vi "Connection Manager (customizable).vi"(9 "Required":cluster{"DI":string[]}[](array[cluster])=[{"DI"=[]}, {"DI"=[]}, {"DI"=["Rep Trigger", "State Change", "Trial Change"]}, {"DI"=["Rep Trigger", "State Change", "Trial Change"]}], 11 "Configuration file":path=path "C:/ProgramData/EPL/Tosca Defaults.ini") -> (2 "Changed":bool)   [LabVIEW 2020]
uses:
  Type Defs/General PXISlot XControl/PXISlotGP.xctl
  Utility VIs/Controls/KListboxEx/KListboxEx.xctl
  Utility VIs/Controls/KTable/KTable.xctl
  Type Defs/CM-Connection.ctl
  Utility VIs/Controls/KTable/Event Type.ctl
  Utility VIs/File IO VIs/Configuration File Wrapper VIs/Config-Read Key (string).vi
  Utility VIs/File IO VIs/Configuration File Wrapper VIs/Config-Write Key (string).vi
  epl-tosca/LV Source/TTL VIs/Device Classes/Base Class/TTLControlledDevice.lvclass
  epl-tosca/LV Source/TTL VIs/Typedefs/TTLControlledDevice XControl/TTLControlledDevice.xctl
  D:/Development/epl-vi-lib/Koop/KObject Class/KObject.lvclass
  D:/Development/epl-tosca/LV Source/TTL VIs/Device Classes/Base Class/TTLControlledDevice.lvclass
  epl-tosca/LV Source/TTL VIs/Device Classes/WaterDelivery Class/TTLWaterDelivery.lvclass
panel:
  in  "Show effectors":bool
  in  "DE List":i32(xcontrol)
  out "read config":bool=TRUE
  in  "DI List":i32(xcontrol) caption="Inputs"
  in  "DO List":i32(xcontrol) caption="Outputs"
  in  "AI List":i32(xcontrol) caption="Inputs"
  in  "AO List":i32(xcontrol)=1 caption="Outputs"
  in  "Apply Button":bool
  in  "Show digital":bool
  in  "Show analog":bool
  out "Save Op":enum16{"None", "Save", "Save and Exit"}(ring)
  in  "Hide unused":bool
  in  "Exit":bool
  in  "Tab Control":enum32{"Analog", "Digital", "Effectors"}(tab)=enum."Effectors"
  in  "Conn2":cluster{"Outputs":string[], "Inputs":string[]}(xcontrol)={"Outputs"=["", ""], "Inputs"=["", "", "", "", "", "", "", ""]} caption="Slot -1"
  in  "Conn1":cluster{"Outputs":string[], "Inputs":string[]}(xcontrol)={"Outputs"=["", ""], "Inputs"=["", ""]} caption="Slot -1"
  in  "Conn3":cluster{"Outputs":string[], "Inputs":string[]}(xcontrol)={"Outputs"=["Fuck", "Freefield"], "Inputs"=["", "", "", "", "", "", "", ""]} caption="Slot -1"
  in  "Conn4":cluster{"Outputs":string[], "Inputs":string[]}(xcontrol)={"Outputs"=["", "", "", ""], "Inputs"=["", "", "", "", "", "", "", ""]} caption="Slot -1"
  in  "Conn5":cluster{"Outputs":string[], "Inputs":string[]}(xcontrol) caption="Slot -1"
  in  "DO Port":u16(ring)=7 caption="Digital Output Port" items=["PXI1Slot6/port0", "PXI1Slot6/port1", "PXI1Slot6/port2", "PXI1Slot7/port0", "PXI1Slot7/port1", "PXI1Slot7/port2", "PXI1Slot8/port0", "PXI1Slot8/port1", "PXI1Slot8/port2"]
  in  "DI Port":u16(ring)=6 caption="Digital Input Port" items=["PXI1Slot6/port0", "PXI1Slot6/port1", "PXI1Slot6/port2", "PXI1Slot7/port0", "PXI1Slot7/port1", "PXI1Slot7/port2", "PXI1Slot8/port0", "PXI1Slot8/port1", "PXI1Slot8/port2"]
  in  "DO Table":u16(xcontrol)
  in  "DI Table":u16(xcontrol)
  in  "DigDevice 4":refnum<class "TTLControlledDevice.lvclass">(xcontrol)
  in  "DigDevice 3":refnum<class "TTLControlledDevice.lvclass">(xcontrol)
  in  "DigDevice 2":refnum<class "TTLControlledDevice.lvclass">(xcontrol)
  in  "DigDevice 1":refnum<class "TTLControlledDevice.lvclass">(xcontrol)=refnum
  in  "DigDevice 0":refnum<class "TTLControlledDevice.lvclass">(xcontrol)=refnum
  # "ANALOG"
  # "DIGITAL"
  # "TTL-Controlled Devices"
  # "DIGITAL"
  # "TTL-Controlled Devices"
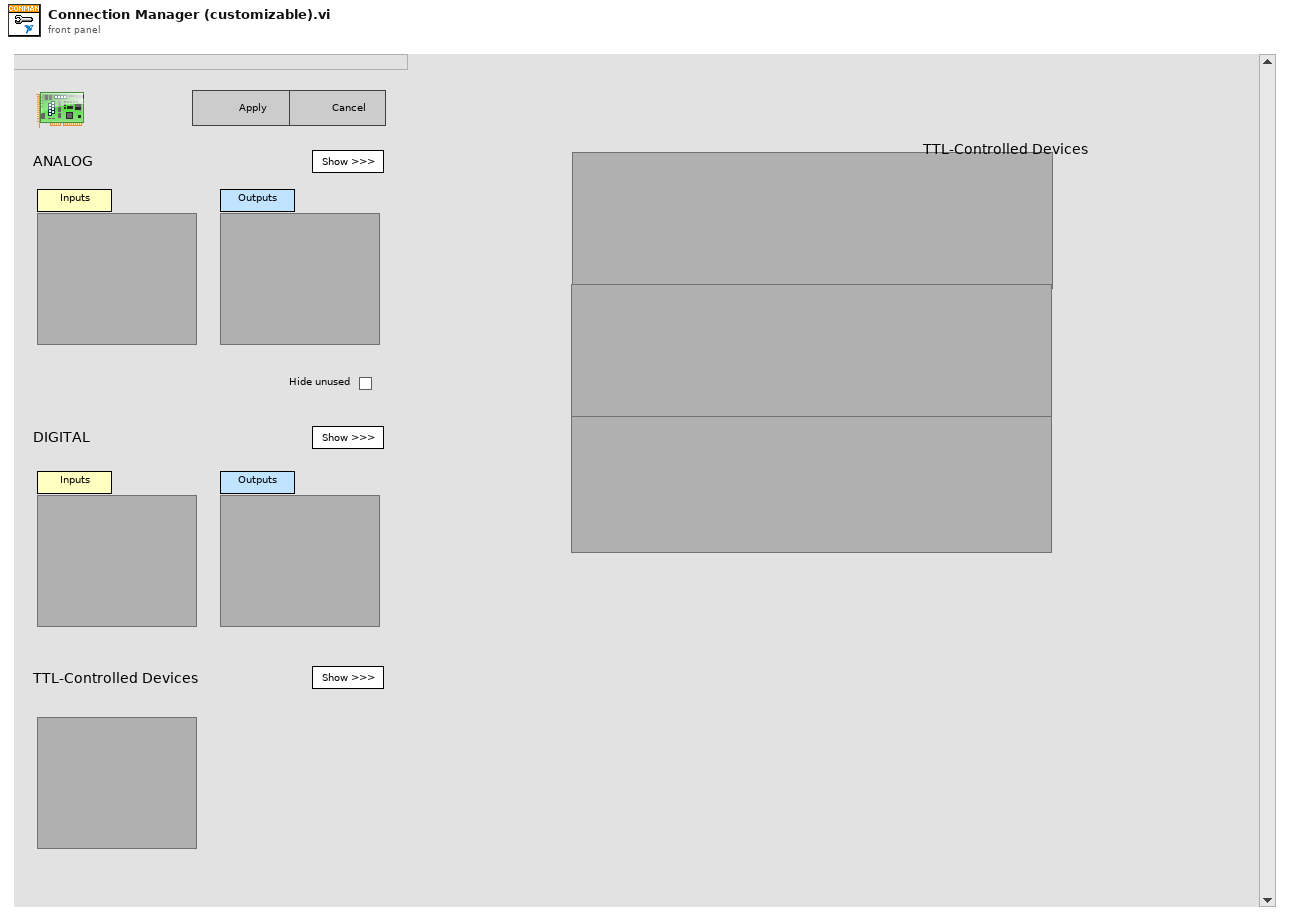
[diagram p1: front panel]
types:
  T1 = typedef "CM-Connection.ctl" = cluster{"IOChannel":string, "Endpoint":string}
  T2 = typedef "KTable.xctl/Event Type.ctl" = enum16{"None", "Selection", "Edit", "Insert", "Delete", "Up", "Down", "Duplicate"}
  T3 = typedef "PXI-Device Spec.ctl" = cluster{"Slot":i32, "ProductType":string, "NumAO":i32, "NumAI":i32, "Device Name":string}
  T4 = cluster{"AO Endpoints":string[], "AI Endpoints":string[]}[]
  T5 = typedef "Connector Type.ctl" = enum16{"None", "PXI-4461", "BNC-2110", "BNC-2090", "PXIe-4463", "PXIe-4464"}
  T6 = typedef "KListboxEx.xctl/Event Action.ctl" = enum16{"None", "Add", "Delete", "Move", "Edit", "Select"}
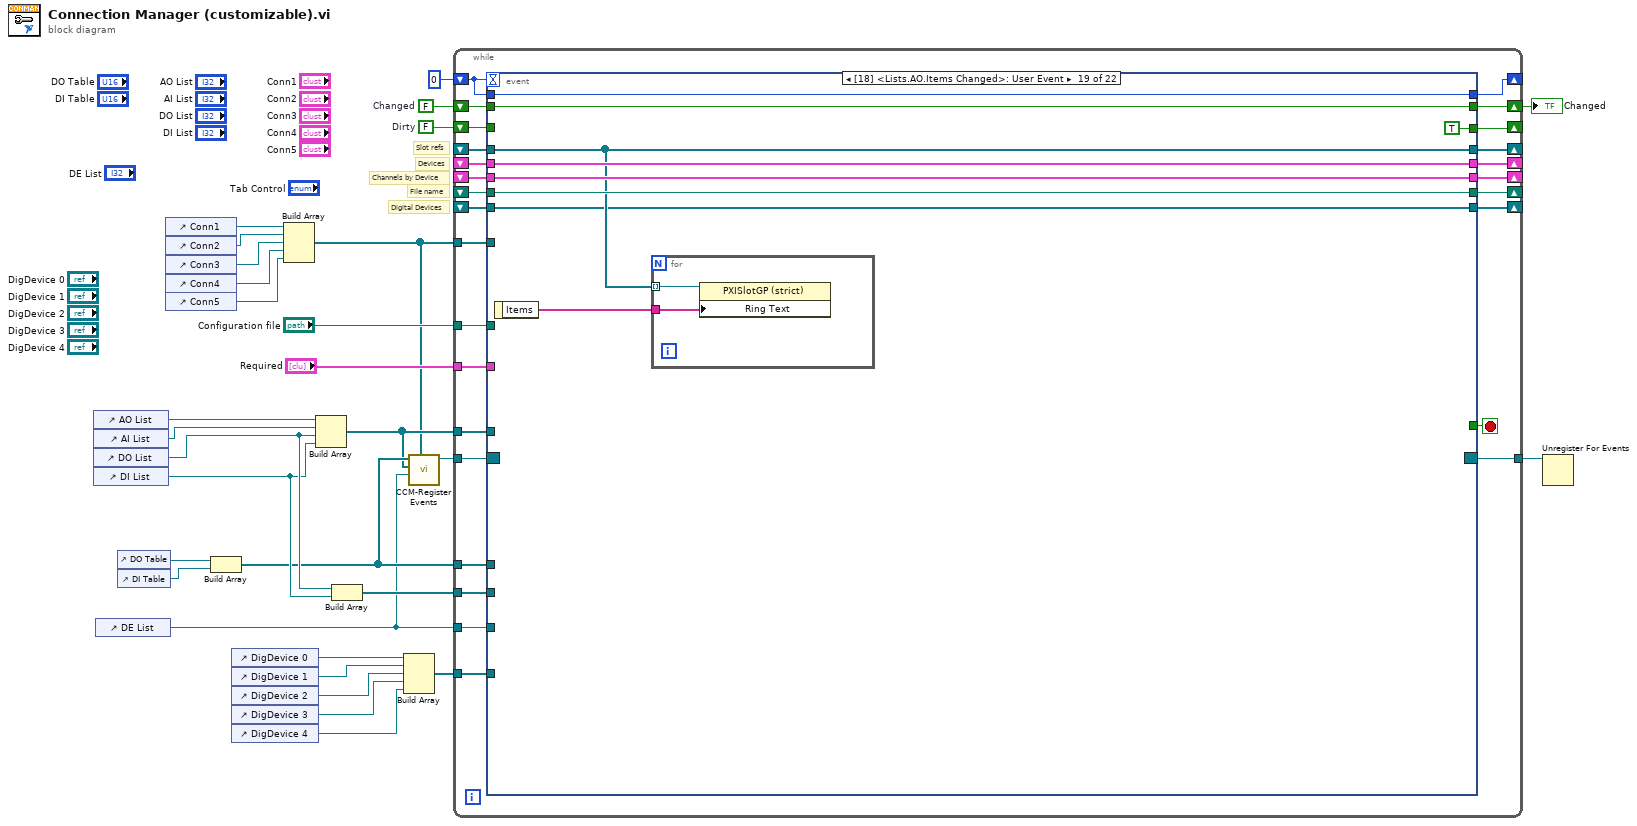
[diagram p0: block diagram]
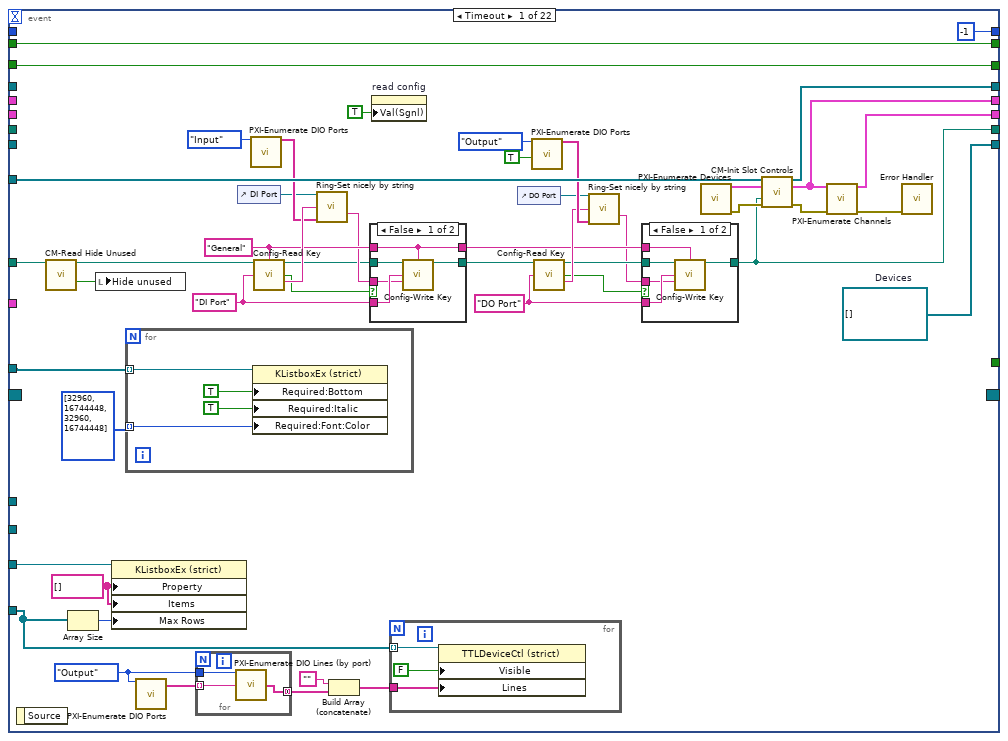
[diagram p2: hidden frame]
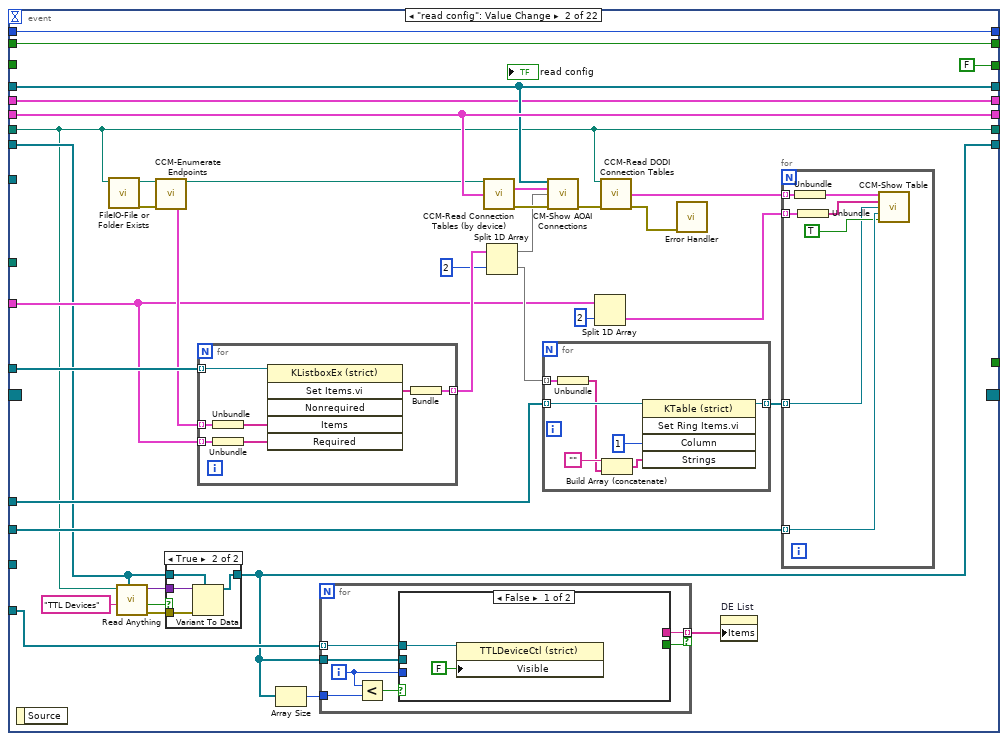
[diagram p5: hidden frame]
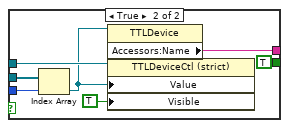
[diagram p6: hidden frame]
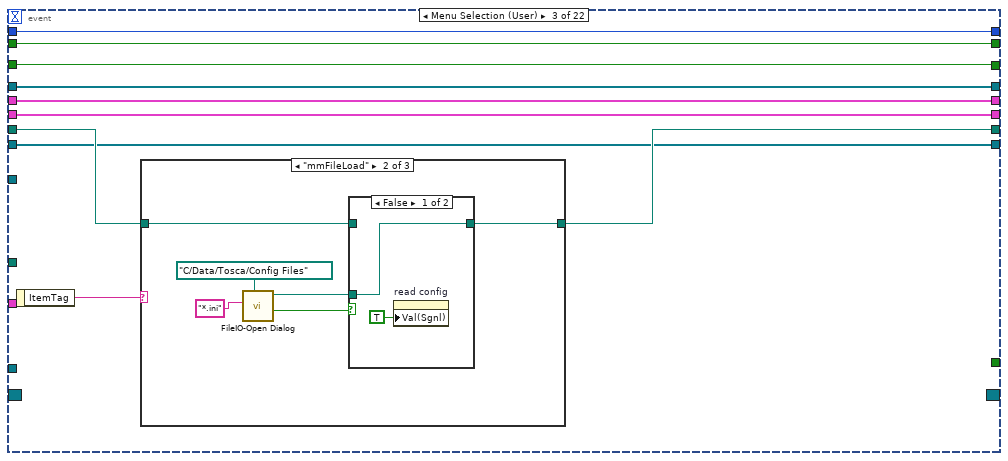
[diagram p8: hidden frame]
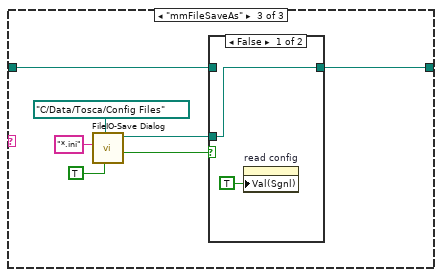
[diagram p11: hidden frame]
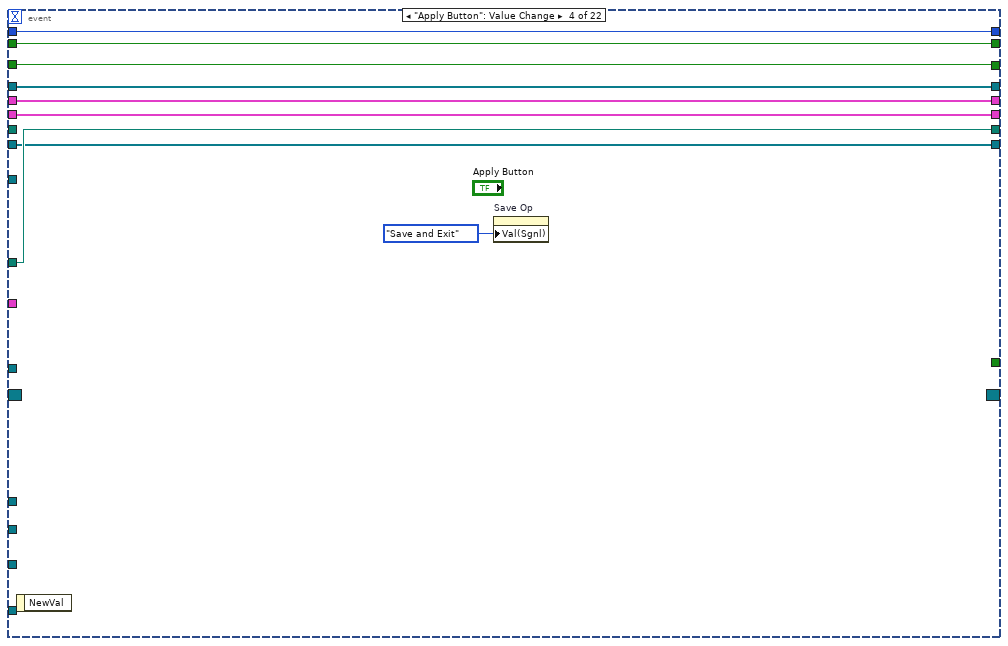
[diagram p13: hidden frame]
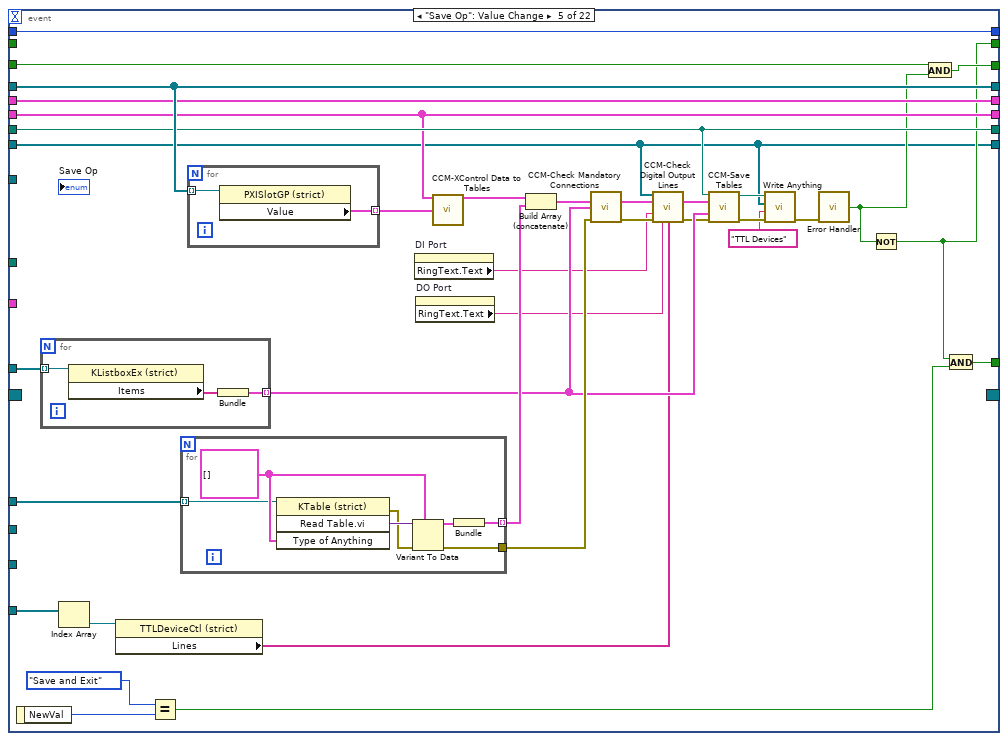
[diagram p14: hidden frame]
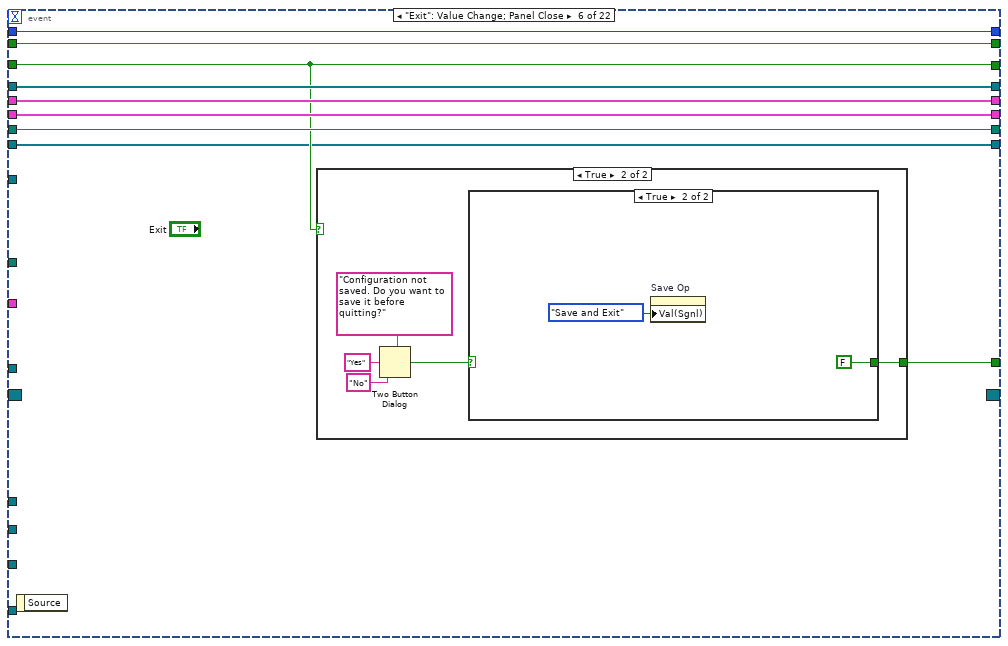
[diagram p15: hidden frame]
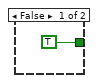
[diagram p16: hidden frame]
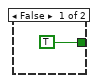
[diagram p17: hidden frame]
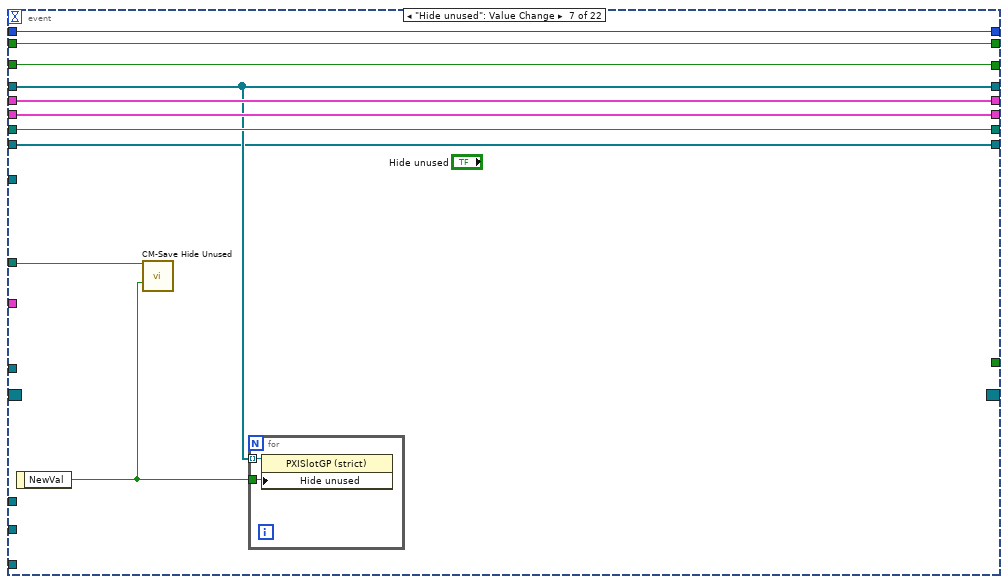
[diagram p18: hidden frame]
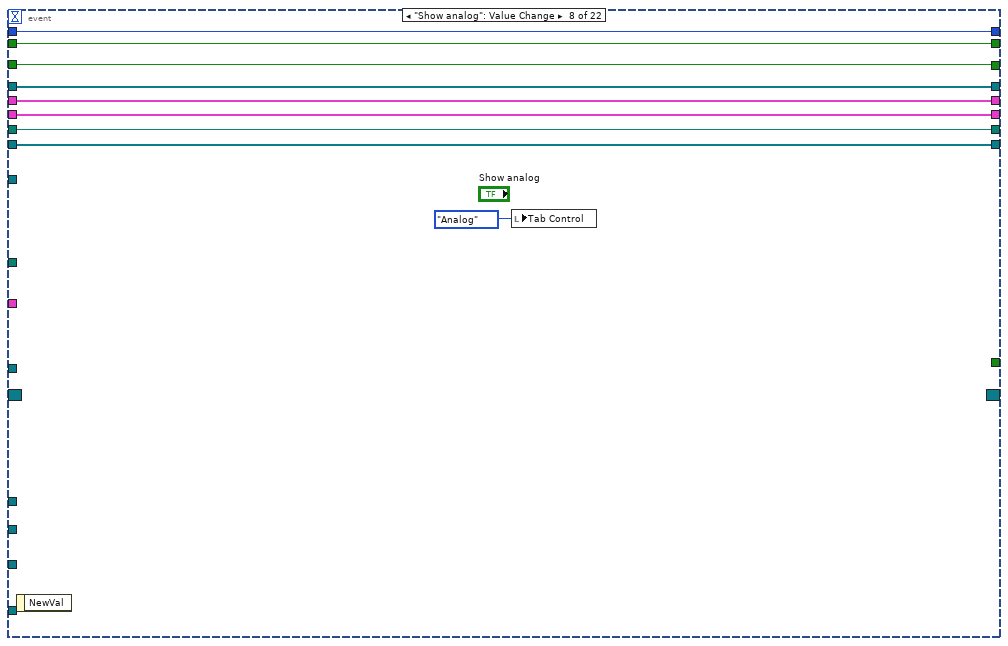
[diagram p19: hidden frame]
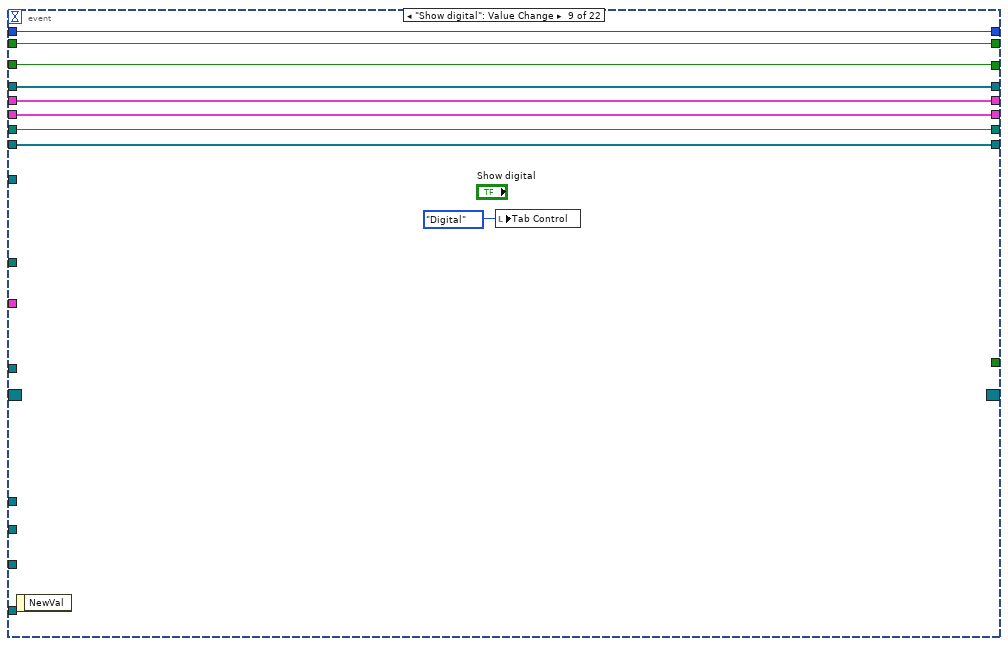
[diagram p20: hidden frame]
diagram:
  w20 = FALSE  # Changed
  w23 = FALSE  # Dirty
  # "Digital Devices"
  # "File name"
  # "Channels by Device"
  # "Devices"
  # "Slot refs"
  n1 = control-ref of="AO List"() -> (w22:refnum<vi>)
  n2 = control-ref of="AI List"() -> (w21:refnum<vi>)
  n3 = control-ref of="DO List"() -> (w19:refnum<vi>)
  n4 = control-ref of="DI List"() -> (w18:refnum<vi>)
  n5 = control-ref of="DE List"() -> (w7:refnum<vi>)
  n6 = control-ref of="DO Table"() -> (w16:refnum<vi>)
  n7 = control-ref of="DI Table"() -> (w15:refnum<vi>)
  n8 = control-ref of="Conn1"() -> (w26:refnum<vi>)
  n9 = control-ref of="Conn2"() -> (w27:refnum<vi>)
  n10 = control-ref of="Conn3"() -> (w28:refnum<vi>)
  n11 = control-ref of="Conn4"() -> (w25:refnum<vi>)
  n12 = control-ref of="Conn5"() -> (w24:refnum<vi>)
  n13 = Build Array(w16, w15) -> (w13:refnum<vi>[])
  n14 = control-ref of="DigDevice 0"() -> (w6:refnum<vi>)
  n15 = control-ref of="DigDevice 1"() -> (w5:refnum<vi>)
  n16 = control-ref of="DigDevice 2"() -> (w3:refnum<vi>)
  n17 = control-ref of="DigDevice 3"() -> (w2:refnum<vi>)
  n18 = control-ref of="DigDevice 4"() -> (w4:refnum<vi>)
  n19 = Build Array(w26, w27, w28, w25, w24) -> (w8:refnum<vi>[])
  n20 = Build Array(w22, w21, w19, w18) -> (w12:refnum<vi>[])
  n21 = Build Array(w19, w18) -> (w17:refnum<vi>[])
  n22 = Build Array(w6, w5, w3, w2, w4) -> (w1:refnum<vi>[])
  n23 = call "CCM-Register Events.vi"("Conn Refs"=w8, "DE List"=w7, "List Refs"=w12, "Table Refs"=w13) -> ("Event Registration Refnum"=w14:refnum<event-registration>)  [unwired: 5 in, 2 out]
  n24 = while {
    shift-right: [w56] -> _
    shift-left: 0 -> [w48]
    shift-right: [w52] -> _
    shift-left: _ -> [w55]
    tunnel: w8 -> [w53]
    shift-right: [w50] -> _
    shift-left: w23 -> [w51]
    tunnel: "Configuration file" -> [w54]
    tunnel: "Required" -> [w49]
    tunnel: w12 -> [w47]
    shift-right: [w46] -> _
    shift-left: _ -> [w45]
    shift-right: [w43] -> w10
    shift-left: w20 -> [w44]
    shift-right: [w42] -> _
    shift-left: _ -> [w41]
    shift-right: [w40] -> _
    shift-left: _ -> [w39]
    tunnel: w17 -> [w38]
    tunnel: w13 -> [w37]
    tunnel: w14 -> [w36]
    tunnel: [w35] -> w11
    tunnel: w7 -> [w34]
    tunnel: w1 -> [w33]
    shift-right: [w32] -> _
    shift-left: _ -> [w31]
    stop <- w57 stop-if-true
    n25 = event shown="[18] <Lists.AO.Items Changed>: User Event" {
      selector: w36 -> [_ _ _ _ _ _ _ _ _ _ _ _ _ _ _ _ _ _ _ _ _ _]
      dyn-events: [_ _ _ _ _ _ _ _ _ _ _ _ _ _ _ _ _ _ _ _ _ _] -> w35
      timeout: w48 -> [_ _ _ _ _ _ _ _ _ _ _ _ _ _ _ _ _ _ _ _ _ _]
      tunnel: [_ _ _ _ w262 w300 _ _ _ _ _ _ _ _ _ _ _ _ _ _ _ _] -> w57
      tunnel: [-1 w161 w208 w238 w272 w294 w312 w324 w333 w349 w361 w369 w407 w433 w445 w457 w469 w481 w490 w501 w517 w586] -> w56
      tunnel: w55 -> [_ w141 w215 w245 w280 w301 w315 w331 w340 w348 w356 w368 w406 w432 w444 w456 w468 w480 w484 w495 w516 w585]
      tunnel: w54 -> [w91 _ _ w239 _ _ w314 _ _ _ w354 _ w400 w426 _ _ _ _ _ _ _ _]
      tunnel: w53 -> [w100 _ _ _ _ _ _ _ _ _ _ _ _ _ _ _ _ _ _ _ _ _]
      tunnel: [w101 w141 w215 w245 w280 w301 w315 w331 w340 w348 w356 w368 w406 w432 w444 w456 w468 w480 w484 w495 w516 w585] -> w52
      tunnel: w51 -> [w98 _ w216 w243 w276 w295 w320 w329 w338 w347 w355 _ w401 w427 w436 w448 _ _ _ _ _ _]
      tunnel: [w98 FALSE w216 w243 w275 w295 w320 w329 w338 w347 w355 TRUE ("Dirty") w401 w427 w435 w447 TRUE ("Dirty") TRUE ("Dirty") TRUE ("Dirty") TRUE ("Dirty") TRUE TRUE ("Dirty")] -> w50
      tunnel: w49 -> [_ w143 _ _ _ _ _ _ _ _ _ _ w385 _ _ _ _ _ _ _ _ _]
      tunnel: w48 -> [_ w161 w208 w238 w272 w294 w312 w324 w333 w349 w361 w369 w407 w433 w445 w457 w469 w481 w490 w501 w517 w586]
      tunnel: w47 -> [w103 w160 _ _ w273 _ _ _ _ _ _ _ _ _ _ _ _ _ _ _ _ _]
      tunnel: [w97 w140 w213 w242 w274 w299 w319 w328 w337 w346 w360 w367 w405 w431 w443 w455 w467 w479 w489 w500 w515 w584] -> w46
      tunnel: w45 -> [_ w140 w213 w242 w274 w299 w319 w328 w337 w346 w360 w367 w405 w431 w443 w455 w467 w479 w489 w500 w515 w584]
      tunnel: w44 -> [w99 w159 w212 w241 _ w298 w318 w327 w336 w345 w359 w366 w404 w430 w442 w454 w466 w478 w488 w499 w504 w574]
      tunnel: [w99 w159 w212 w241 w260 w298 w318 w327 w336 w345 w359 w366 w404 w430 w442 w454 w466 w478 w488 w499 w504 w574] -> w43
      tunnel: [w96 w155 w211 w240 w270 w297 w317 w326 w335 w344 w358 w365 w403 w429 w441 w453 w465 w477 w487 w498 w514 w583] -> w42
      tunnel: w41 -> [_ w155 w211 w240 w270 w297 w317 w326 w335 w344 w358 w365 w403 w429 w441 w453 w465 w477 w487 w498 w514 w583]
      tunnel: [w70 w133 w209 w239 w271 w296 w316 w325 w334 w343 w357 w364 w402 w428 w440 w452 w464 w476 w486 w497 w513 w582] -> w40
      tunnel: w39 -> [_ w133 w210 _ w271 w296 w316 w325 w334 w343 w357 w364 w402 w428 w440 w452 w464 w476 w486 w497 w513 w582]
      tunnel: w38 -> [_ w149 _ _ _ _ _ _ _ _ _ _ w383 _ _ _ _ _ _ _ _ _]
      tunnel: w37 -> [_ w147 _ _ w267 _ _ _ _ _ _ _ w384 _ _ _ _ _ _ _ _ _]
      tunnel: w34 -> [w67 _ _ _ _ _ _ _ _ _ _ _ _ _ _ _ _ _ _ _ _ _]
      tunnel: w33 -> [w64 w132 _ _ w252 _ _ _ _ _ _ _ _ _ _ _ _ _ _ _ w512 w580]
      tunnel: [w63 w130 w207 w237 w253 w293 w311 w323 w332 w341 w350 w362 w398 w423 w434 w446 w458 w470 w482 w493 w507 w578] -> w32
      tunnel: w31 -> [_ w135 w207 w237 w253 w293 w311 w323 w332 w341 w350 w362 w398 w423 w434 w446 w458 w470 w482 w493 w508 w581]
      event Timeout {
        w61 = enum16{"Input", "Output"}."Output" ("Direction")
        w63 = refnum<class "TTLControlledDevice.lvclass">[] []  # Devices
        w66 = string[] [] ("Items")
        w71 = "DO Port" ("key")
        w77 = "DI Port" ("key")
        w78 = "General" ("section")
        n26 = event-data() -> ()  [unwired: 1 in, 1 out]
        n27 = call "CM-Read Hide Unused.vi"("configuration file path"=w91) -> ("file path"=w90:path, "Hide unused"=w89:bool)  [unwired: 12 in, 1 out]
        n28 = Array Size(array=w64) -> (size(s)=w65:i32)
        n29 = local write "Hide unused"(w89) -> ()
        n30 = property class="KListboxEx (strict)"(reference=w67, "Property"=w66, "Items"=w66, "Max Rows"=w65) -> ()  [unwired: 1 in, 2 out]
        n31 = for {
          tunnel: w103 -> [w126] mode=indexing
          tunnel: u32[] [32960, 16744448, 32960, 16744448] -> [w125] mode=indexing
          n32 = property class="KListboxEx (strict)"(reference=w126, "Required:Bottom"=TRUE, "Required:Italic"=TRUE ("Required:Font:Italic"), "Required:Font:Color"=w125) -> ()  [unwired: 1 in, 2 out]
        }
        n33 = call "PXI-Enumerate DIO Ports.vi"("Direction"=w61) -> ("Ports"=w62:tag[])  [unwired: 13 in, 1 out]
        n34 = for {
          tunnel: w62 -> [w107] mode=indexing
          tunnel: w61 -> [w108]
          tunnel: [w106] -> w60 mode=concatenating
          n35 = call "PXI-Enumerate DIO Lines (by port).vi"("Direction"=w108, "Port"=w107) -> ("Dev/Port/Lines"=w106:tag[])  [unwired: 11 in, 2 out]
        }
        n36 = control-ref of="DI Port"() -> (w83:refnum<vi>)
        n37 = call "PXI-Enumerate DIO Ports.vi"("Direction"=enum16{"Input", "Output"}."Input") -> ("Ports"=w84:tag[])  [unwired: 13 in, 1 out]
        n38 = call-poly "Config-Read Key.vi"("configuration file path"=w90, "section"=w78, "key"=w77) -> ("file path"=w75:path, "found?"=w79:bool, "value"=w85:string)  [unwired: 9 in, 1 out]
        n39 = call "Ring-Set nicely by string.vi"("Ring in"=w83, "Device"=w85, "Strings []"=w84) -> ("Selection"=w76:string)  [unwired: 8 in, 4 out]
        n40 = Build Array (concatenate)("", w60) -> (w59:string[])
        n41 = case shown="False" w79 {
          tunnel: w78 -> [w120 w124]
          tunnel: w77 -> [w122 _]
          tunnel: w76 -> [w121 _]
          tunnel: [w120 w124] -> w73
          tunnel: w75 -> [w119 w123]
          tunnel: [w118 w123] -> w74
          frame False {
            n42 = call-poly "Config-Write Key.vi"("configuration file path"=w119, "section"=w120, "key"=w122, "value"=w121) -> ("file path"=w118:path)  [unwired: 9 in, 2 out]
          }
          frame True {
          }
        }
        n43 = property on="read config" class="Bool (strict)"("Val(Sgnl)"=TRUE ("Value (Signaling)")) -> ()  [unwired: 2 in, 2 out]
        n44 = for {
          tunnel: w64 -> [w111] mode=indexing
          tunnel: w59 -> [w109]
          n45 = property class="TTLDeviceCtl (strict)"(reference=w111, "Visible"=FALSE, "Lines"=w109) -> ()  [unwired: 1 in, 2 out]
        }
        n46 = control-ref of="DO Port"() -> (w81:refnum<vi>)
        n47 = call "PXI-Enumerate DIO Ports.vi"("Direction"=enum16{"Input", "Output"}."Output", "Must be buffered"=TRUE) -> ("Ports"=w82:tag[])  [unwired: 12 in, 1 out]
        n48 = call-poly "Config-Read Key.vi"("configuration file path"=w74, "key"=w71) -> ("file path"=w72:path, "found?"=w68:bool, "value"=w80:string)  [unwired: 10 in, 1 out]
        n49 = call "Ring-Set nicely by string.vi"("Ring in"=w81, "Device"=w80, "Strings []"=w82) -> ("Selection"=w69:string)  [unwired: 8 in, 4 out]
        n50 = case shown="False" w68 {
          tunnel: w73 -> [w114 _]
          tunnel: w71 -> [w116 _]
          tunnel: w69 -> [w115 _]
          tunnel: w72 -> [w113 w117]
          tunnel: [w112 w117] -> w70
          frame False {
            n51 = call-poly "Config-Write Key.vi"("configuration file path"=w113, "section"=w114, "key"=w116, "value"=w115) -> ("file path"=w112:path)  [unwired: 9 in, 2 out]
          }
          frame True {
          }
        }
        n52 = call "PXI-Enumerate Devices.vi"() -> ("Devices"=w102:T3[], "error out"=w95:errorcluster)  [unwired: 14 in]
        n53 = call "CM-Init Slot Controls.vi"("slot ctl refs"=w100, "Devices"=w102, "config file"=w70, "error in (no error)"=w95) -> ("slot ctl refs out"=w101:refnum<vi>[], "Devices thru"=w97:T3[], "error out"=w94:errorcluster)  [unwired: 9 in]
        n54 = call "PXI-Enumerate Channels.vi"("Devices"=w97, "error in (no error)"=w94) -> ("Channels By Device"=w96:cluster{"Out":string[], "In":string[]}[], "error out"=w93:errorcluster)  [unwired: 11 in, 1 out]
        n55 = call "Error Handler.vi"("error in (no error)"=w93) -> ()  [unwired: 13 in, 2 out]
      }
      event "read config": Value Change {
        n56 = event-data() -> ()  [unwired: 1 in, 1 out]
        n57 = call "FileIO-File or Folder Exists.vi"("path"=w133) -> ("error out"=w163:errorcluster, "dup path"=w164:path)  [unwired: 7 in, 2 out]
        n58 = call "Read Anything.vi"("Type of Anything"=w135, "Section Name (Name of \"Type of Anything\")"="TTL Devices" ("Section Name (Name of \"Type of Anything\")"), "Path (dialog)"=w133) -> ("Error Out"=w137:errorcluster, "Found?"=w134:bool, "Anything"=w136:variant)  [unwired: 6 in]
        n59 = call "CCM-Enumerate Endpoints.vi"("Path In"=w164, "error in (no error)"=w163) -> ("Path Out"=w139:path, "Endpoints"=w158:cluster{"Name":string[]}[])  [unwired: 9 in, 3 out]
        n60 = case shown="True" w134 {
          tunnel: w137 -> [_ w185]
          tunnel: w136 -> [_ w184]
          tunnel: w135 -> [w181 w183]
          tunnel: [w181 w182] -> w130
          frame False {
          }
          frame True {
            n61 = Variant To Data(error in=w185, type=w183, Variant=w184) -> (data=w182:refnum<class "TTLControlledDevice.lvclass">[])  [unwired: 1 out]
          }
        }
        n62 = for {
          tunnel: w158 -> [w205] mode=indexing
          tunnel: w160 -> [w206] mode=indexing
          tunnel: w143 -> [w203] mode=indexing
          tunnel: [w200] -> w157 mode=indexing
          n63 = Unbundle(w205) -> ("Name"=w204:string[])
          n64 = Unbundle(w203) -> ("DI"=w202:string[])
          n65 = invoke on="Invoke Node" class="KListboxEx (strict)" method="Set Items.vi"(reference=w206, "Items"=w204, "Required"=w202) -> ("Set Items.vi"=w201:string[])  [unwired: 3 in, 5 out]
          n66 = Bundle("Set Items.vi"=w201) -> (w200:cluster{"Set Items.vi":string[]})  [unwired: 1 in]
        }
        n67 = Array Size(array=w130) -> (size(s)=w131:i32)
        n68 = for {
          tunnel: w132 -> [w169] mode=indexing
          tunnel: w131 -> [w171]
          tunnel: w130 -> [w167]
          tunnel: [w166] -> w129 mode=indexing if=w165
          i -> [w168]
          n69 = Less?(x=w168, y=w171) -> (x < y?=w170:bool)
          n70 = case shown="False" w170 {
            tunnel: w169 -> [w173 w180]
            tunnel: w168 -> [_ w179]
            tunnel: w167 -> [_ w178]
            tunnel: [_ w175] -> w166
            tunnel: [_ TRUE] -> w165
            frame False {
              n71 = property class="TTLDeviceCtl (strict)"(reference=w173, "Visible"=FALSE) -> ()  [unwired: 1 in, 2 out]
            }
            frame True {
              n72 = Index Array(array=w178, index=w179) -> (element=w176:refnum<class "TTLControlledDevice.lvclass">)
              n73 = property class="TTLDevice"(reference=w176) -> ("Accessors:Name"=w175:string)  [unwired: 1 in, 2 out]
              n74 = property class="TTLDeviceCtl (strict)"(reference=w180, "Value"=w176, "Visible"=TRUE) -> ()  [unwired: 1 in, 2 out]
            }
          }
        }
        n75 = call "CCM-Read Connection Tables (by device).vi"("Path In"=w139, "Channels By Device"=w155) -> ("Tables By Device"=w153:T4, "error out"=w154:errorcluster)  [unwired: 11 in, 1 out]
        n76 = Split 1D Array(array=w157, index=2) -> (first subarray=w152:cluster{"Set Items.vi":string[]}[], second subarray=w146:cluster{"Set Items.vi":string[]}[])
        n77 = for {
          tunnel: w147 -> [w189] mode=indexing
          tunnel: w146 -> [w188] mode=indexing
          tunnel: [w186] -> w145 mode=indexing
          n78 = Unbundle(w188) -> ("Set Items.vi"=w187:string[])
          n79 = Build Array (concatenate)("", w187) -> (w191:string[])
          n80 = invoke on="Invoke Node" class="KTable (strict)" method="Set Ring Items.vi"(reference=w189, "Column"=1, "Strings"=w191) -> (reference out=w186:refnum<vi>)  [unwired: 2 in, 4 out]
        }
        n81 = call "CM-Show AOAI Connections.vi"("slot ctl refs"=w141, "Tables By Device"=w153, "Endpoints"=w152, "error in (no error)"=w154) -> ("error out"=w151:errorcluster)  [unwired: 10 in, 1 out]
        n82 = Split 1D Array(array=w143, index=2) -> (second subarray=w142:cluster{"DI":string[]}[])  [unwired: 1 out]
        n83 = call "CCM-Read DODI Connection Tables.vi"("Path In"=w133, "error in (no error)"=w151) -> ("Tables"=w150:cluster{"Table":T1[]}[], "error out"=w148:errorcluster)  [unwired: 11 in, 1 out]
        n84 = call "Error Handler.vi"("error in (no error)"=w148) -> ()  [unwired: 13 in, 2 out]
        n85 = property on="DE List" class="KListboxEx (strict)"("Items"=w129) -> ()  [unwired: 2 in, 2 out]
        n86 = for {
          tunnel: w150 -> [w197] mode=indexing
          tunnel: w142 -> [w196] mode=indexing
          tunnel: w149 -> [w195] mode=indexing
          tunnel: w145 -> [w193] mode=indexing
          n87 = Unbundle(w197) -> ("Table"=w198:T1[])
          n88 = Unbundle(w196) -> ("DI"=w199:string[])
          n89 = call "CCM-Show Table.vi"("Table"=w198, "Required"=w199, "Table Ref"=w193, "List Ref"=w195, "Force required"=TRUE) -> ()  [unwired: 11 in]
        }
      }
      event Menu Selection (User) {
        n90 = event-data() -> ("ItemTag"=w214:string)  [unwired: 1 in]
        n91 = case shown="\"mmFileLoad\"" w214 {
          tunnel: w210 -> [w217 w219 w228]
          tunnel: [w217 w218 w227] -> w209
          frame "False", Default {
          }
          frame "mmFileLoad" {
            n92 = call "FileIO-Open Dialog.vi"("Default Folder"=path "C:/Data/Tosca/Config Files", "pattern (all files)"="*.ini") -> ("cancelled"=w221:bool, "selected path"=w220:path)  [unwired: 7 in, 1 out]
            n93 = case shown="False" w221 {
              tunnel: w220 -> [w225 _]
              tunnel: w219 -> [_ w226]
              tunnel: [w225 w226] -> w218
              frame False {
                n94 = property on="read config" class="Bool (strict)"("Val(Sgnl)"=TRUE ("Value (Signaling)")) -> ()  [unwired: 2 in, 2 out]
              }
              frame True {
              }
            }
          }
          frame "mmFileSaveAs" {
            n95 = call "FileIO-Save Dialog.vi"("Overwrite prompt?"=TRUE, "Default Folder"=path "C:/Data/Tosca/Config Files", "pattern (all files)"="*.ini") -> ("cancelled"=w230:bool, "selected path"=w229:path)  [unwired: 6 in, 1 out]
            n96 = case shown="False" w230 {
              tunnel: w229 -> [w234 _]
              tunnel: w228 -> [_ w236]
              tunnel: [w234 w236] -> w227
              frame False {
                n97 = property on="read config" class="Bool (strict)"("Val(Sgnl)"=TRUE ("Value (Signaling)")) -> ()  [unwired: 2 in, 2 out]
              }
              frame True {
              }
            }
          }
        }
      }
      event "Apply Button": Value Change {
        n98 = event-data() -> ()  [unwired: 1 in, 1 out]
        n99 = property on="Save Op" class="Enum (strict)"("Val(Sgnl)"=enum16{"None", "Save", "Save and Exit"}."Save and Exit" ("Value (Signaling)")) -> ()  [unwired: 2 in, 2 out]
      }
      event "Save Op": Value Change {
        n100 = event-data() -> ("NewVal"=w279:enum16{"None", "Save", "Save and Exit"})  [unwired: 1 in]
        n101 = for {
          tunnel: w273 -> [w290] mode=indexing
          tunnel: [w288] -> w263 mode=indexing
          n102 = property class="KListboxEx (strict)"(reference=w290) -> ("Items"=w289:string[])  [unwired: 1 in, 2 out]
          n103 = Bundle("Items"=w289) -> (w288:cluster{"Items":string[]})  [unwired: 1 in]
        }
        n104 = Index Array(array=w252) -> (element=w251:refnum<vi>)  [unwired: 1 in]
        n105 = property class="TTLDeviceCtl (strict)"(reference=w251) -> ("Lines"=w248:string[])  [unwired: 1 in, 2 out]
        n106 = Equal?(x=enum16{"None", "Save", "Save and Exit"}."Save and Exit", y=w279) -> (x = y?=w277:bool)
        n107 = for {
          tunnel: [w282] -> w265 mode=indexing
          tunnel: w267 -> [w281] mode=indexing
          tunnel: [w285] -> w264
          w284 = T1[] []
          n108 = invoke on="Invoke Node" class="KTable (strict)" method="Read Table.vi"(reference=w281, "Type of Anything"=w284) -> (error out=w286:errorcluster, "Read Table.vi"=w287:variant)  [unwired: 2 in, 2 out]
          n109 = Variant To Data(error in=w286, type=w284, Variant=w287) -> (data=w283:T1[], error out=w285:errorcluster)
          n110 = Bundle(w283) -> (w282:cluster{T1[]})  [unwired: 1 in]
        }
        n111 = for {
          tunnel: w280 -> [w292] mode=indexing
          tunnel: [w291] -> w268 mode=indexing
          n112 = property class="PXISlotGP (strict)"(reference=w292) -> ("Value"=w291:cluster{"Outputs":string[], "Inputs":string[]})  [unwired: 1 in, 2 out]
        }
        n113 = property on="DI Port" class="Ring (strict)"() -> ("RingText.Text"=w246:string)  [unwired: 2 in, 2 out]
        n114 = property on="DO Port" class="Ring (strict)"() -> ("RingText.Text"=w249:string)  [unwired: 2 in, 2 out]
        n115 = call "CCM-XControl Data to Tables.vi"("Channels By Device"=w270, "Endpoints by Channel by Device"=w268) -> ("Tables"=w269:cluster{"Table":T1[]}[])  [unwired: 13 in]
        n116 = Build Array (concatenate)(w269, w265) -> (w266:cluster{"Table":T1[]}[])
        n117 = call "CCM-Check Mandatory Connections.vi"("Tables"=w266, "Mandatory"=w263, "error in (no error)"=w264) -> ("Tables thru"=w250:cluster{"Table":T1[]}[], "error out"=w255:errorcluster)  [unwired: 11 in]
        n118 = call "CCM-Check Digital Output Lines.vi"("TTL Devices"=w253, "Tables"=w250, "DI Port"=w246, "error in (no error)"=w255, "Buffered DO Port"=w249, "DO Lines"=w248) -> ("Tables thru"=w247:cluster{"Table":T1[]}[], "error out"=w254:errorcluster)  [unwired: 8 in]
        n119 = call "CCM-Save Tables.vi"("configuration file path"=w271, "Tables"=w247, "Endpoints"=w263, "error in (no error)"=w254) -> ("file path"=w257:path, "error out"=w258:errorcluster)  [unwired: 10 in]
        n120 = call "Write Anything.vi"("Error In"=w258, "Section Name (Name of \"Anything\")"="TTL Devices" ("Section Name (Name of \"Anything\")"), "Anything"=w253, "Path (dialog)"=w257) -> ("Error Out"=w259:errorcluster)  [unwired: 6 in, 1 out]
        n121 = call "Error Handler.vi"("error in (no error)"=w259) -> ("error?"=w261:bool)  [unwired: 13 in, 1 out]
        n122 = Not(x=w261) -> (.not. x?=w260:bool)
        n123 = And(x=w276, y=w261) -> (x .and. y?=w275:bool)
        n124 = And(x=w260, y=w277) -> (x .and. y?=w262:bool)
      }
      event "Exit": Value Change; Panel Close {
        n125 = event-data() -> ()  [unwired: 1 in, 1 out]
        n126 = case shown="True" w295 {
          tunnel: [TRUE w303] -> w300
          frame False {
          }
          frame True {
            n127 = Two Button Dialog(message="Configuration not saved. Do you want to save it before quitting?", 1:"No" ("F button name (\"Cancel\")"), 2:"Yes" ("T button name (\"OK\")")) -> (T button?=w304:bool)
            n128 = case shown="True" w304 {
              tunnel: [TRUE FALSE] -> w303
              frame False {
              }
              frame True {
                n129 = property on="Save Op" class="Enum (strict)"("Val(Sgnl)"=enum16{"None", "Save", "Save and Exit"}."Save and Exit" ("Value (Signaling)")) -> ()  [unwired: 2 in, 2 out]
              }
            }
          }
        }
      }
      event "Hide unused": Value Change {
        n130 = event-data() -> ("NewVal"=w313:bool)  [unwired: 1 in]
        n131 = call "CM-Save Hide Unused.vi"("configuration file path"=w314, "Hide unused"=w313) -> ()  [unwired: 12 in, 2 out]
        n132 = for {
          tunnel: w315 -> [w322] mode=indexing
          tunnel: w313 -> [w321]
          n133 = property class="PXISlotGP (strict)"(reference=w322, "Hide unused"=w321) -> ()  [unwired: 1 in, 2 out]
        }
      }
      event "Show analog": Value Change {
        n134 = event-data() -> ()  [unwired: 1 in, 1 out]
        n135 = local write "Tab Control"(enum32{"Analog", "Digital"}."Analog" ("Tab Control")) -> ()
      }
      event "Show digital": Value Change {
        n136 = event-data() -> ()  [unwired: 1 in, 1 out]
        n137 = local write "Tab Control"(enum32{"Analog", "Digital"}."Digital" ("Tab Control")) -> ()
      }
      event "Show effectors": Value Change {
        n138 = event-data() -> ()  [unwired: 1 in, 1 out]
        n139 = local write "Tab Control"(enum32{"Analog", "Digital", "Effectors"}."Effectors" ("Tab Control")) -> ()
      }
      event User Event {
        n140 = event-data() -> ("Device"=w353:string, "ConType"=w352:T5)  [unwired: 1 in]
        n141 = call "CM-Save Connector Type.vi"("configuration file path"=w354, "Device"=w353, "ConType"=w352) -> ("error out"=w351:errorcluster)  [unwired: 11 in, 1 out]
        n142 = call "CM-Layout Slot Controls.vi"("SlotRefs"=w356, "error in (no error)"=w351) -> ()  [unwired: 13 in, 1 out]
      }
      event "Conn1", "Conn2", "Conn3", "Conn4", "Conn5": Value Change {
        n143 = event-data() -> ()  [unwired: 1 in, 1 out]
      }
      event "DI Port": Value Change {
        w382 = 1 ("index")
        w389 = T1[] []
        n144 = event-data() -> ()  [unwired: 1 in, 1 out]
        n145 = property on="DI Port" class="Ring (strict)"() -> ("RingText.Text"=w388:string)  [unwired: 2 in, 2 out]
        n146 = Index Array(array=w384, index=w382) -> (element=w374:refnum<vi>)
        n147 = Index Array(array=w383, index=w382) -> (element=w371:refnum<vi>)
        n148 = Index Array(array=w385, index=3) -> (element=w380:cluster{"DI":string[]})
        n149 = call-poly "Config-Write Key.vi"("configuration file path"=w400, "key"="DI Port", "value"=w388) -> ("error out"=w397:errorcluster)  [unwired: 10 in, 2 out]
        n150 = invoke on="DI Table" class="KTable (strict)" method="Read Table.vi"(error in=w397, "Type of Anything"=w389) -> ("Read Table.vi"=w396:variant)  [unwired: 2 in, 3 out]
        n151 = call "PXI-Enumerate DIO Lines (by port).vi"("Direction"=enum16{"Input", "Output"}."Input", "Port"=w388) -> ("Lines"=w390:string[])  [unwired: 11 in, 2 out]
        n152 = property class="KListboxEx (strict)"(reference=w371) -> (reference out=w370:refnum<vi>, "Items"=w372:string[])  [unwired: 1 in, 1 out]
        n153 = Variant To Data(type=w389, Variant=w396) -> (data=w395:T1[])  [unwired: 1 in, 1 out]
        n154 = Array Size(array=w390) -> (size(s)=w392:i32)
        n155 = Array Size(array=w395) -> (size(s)=w393:i32)
        n156 = Less?(x=w392, y=w393) -> (x < y?=w394:bool)
        n157 = case shown="False" w394 {
          tunnel: w395 -> [w417 w422]
          tunnel: w393 -> [w415 w421]
          tunnel: w392 -> [w416 w420]
          tunnel: [w412 w418] -> w391
          frame False {
            n158 = Subtract(x=w416, y=w415) -> (x-y=w414:i32)
            n159 = Initialize Array(T1 {"IOChannel"="", "Endpoint"=""} ("Connection"), w414) -> (w411:T1[])
            n160 = Build Array (concatenate)(w417, w411) -> (w412:T1[])
          }
          frame True {
            n161 = Subtract(x=w421, y=w420) -> (x-y=w419:i32)
            n162 = Delete From Array(array=w422, length=w419, index=w420) -> (array with subset deleted=w418:T1[])  [unwired: 1 out]
          }
        }
        n163 = Build Array (concatenate)("", w372) -> (w376:string[])
        n164 = invoke on="Invoke Node" class="KTable (strict)" method="Set Ring Items.vi"(reference=w374, "Column"=1, "Strings"=w376) -> (reference out=w373:refnum<vi>)  [unwired: 2 in, 4 out]
        n165 = for {
          tunnel: w391 -> [w410] mode=indexing
          tunnel: w390 -> [w408] mode=indexing
          tunnel: [w409] -> w386 mode=indexing
          n166 = Bundle By Name(cluster=w410, "IOChannel"=w408) -> (w409:T1)
        }
        n167 = Unbundle(w380) -> ("DI"=w379:string[])
        n168 = call "CCM-Show Table.vi"("Table"=w386, "Required"=w379, "Table Ref"=w373, "List Ref"=w370, "Force required"=TRUE) -> ()  [unwired: 11 in]
      }
      event "DO Port": Value Change {
        n169 = event-data() -> ()  [unwired: 1 in, 1 out]
        n170 = property on="DO Port" class="Ring (strict)"() -> ("RingText.Text"=w424:string)  [unwired: 2 in, 2 out]
        n171 = call-poly "Config-Write Key.vi"("configuration file path"=w426, "key"="DO Port", "value"=w424) -> ()  [unwired: 10 in, 3 out]
      }
      event User Event {
        n172 = event-data() -> ("Type"=w437:T2)  [unwired: 1 in]
        n173 = Equal?(x=w437, y=Event_Type."Edit") -> (x = y?=w439:bool)
        n174 = Or(x=w436, y=w439) -> (x .or. y?=w435:bool)
      }
      event User Event {
        n175 = event-data() -> ("Type"=w449:T2)  [unwired: 1 in]
        n176 = Equal?(x=w449, y=Event_Type."Edit") -> (x = y?=w451:bool)
        n177 = Or(x=w448, y=w451) -> (x .or. y?=w447:bool)
      }
      event User Event {
        n178 = event-data() -> ()  [unwired: 1 in, 1 out]
        n179 = property on="DO List" class="KListboxEx (strict)"() -> ("Nonrequired"=w463:string[])  [unwired: 2 in, 2 out]
        n180 = Build Array (concatenate)("", w463) -> (w461:string[])
        n181 = invoke on="DO Table" class="KTable (strict)" method="Set Ring Items.vi"("Column"=1, "Strings"=w461) -> ()  [unwired: 3 in, 5 out]
      }
      event User Event {
        n182 = event-data() -> ()  [unwired: 1 in, 1 out]
        n183 = property on="DI List" class="KListboxEx (strict)"() -> ("Nonrequired"=w475:string[])  [unwired: 2 in, 2 out]
        n184 = Build Array (concatenate)("", w475) -> (w473:string[])
        n185 = invoke on="DI Table" class="KTable (strict)" method="Set Ring Items.vi"("Column"=1, "Strings"=w473) -> ()  [unwired: 3 in, 5 out]
      }
      event User Event {
        n186 = event-data() -> ("Items"=w485:string[])  [unwired: 1 in]
        n187 = for {
          tunnel: w484 -> [w492] mode=indexing
          tunnel: w485 -> [w491]
          n188 = property class="PXISlotGP (strict)"(reference=w492, "Ring Text"=w491) -> ()  [unwired: 1 in, 2 out]
        }
      }
      event User Event {
        n189 = event-data() -> ("Items"=w496:string[])  [unwired: 1 in]
        n190 = for {
          tunnel: w495 -> [w503] mode=indexing
          tunnel: w496 -> [w502]
          n191 = property class="PXISlotGP (strict)"(reference=w503, "Input List"=w502) -> ()  [unwired: 1 in, 2 out]
        }
      }
      event User Event {
        n192 = event-data() -> ("Action"=w511:T6, "Name"=w509:string, "Start row"=w510:i32, "End row"=w506:i32)  [unwired: 1 in]
        n193 = case shown="\"Move\"" w511 {
          tunnel: w512 -> [_ w520 w538 w560 w571]
          tunnel: w510 -> [_ w522 w540 w559 w565]
          tunnel: w509 -> [_ w524 _ _ w573]
          tunnel: w508 -> [w518 w526 w541 w561 w566]
          tunnel: [w518 w519 w537 w557 w570] -> w507
          tunnel: w506 -> [_ _ _ w554 _]
          frame "None", Default {
          }
          frame "Add" {
            n194 = property class="TTLDevice"(reference=refnum<class "TTLControlledDevice.lvclass"> refnum ("DigEffDevice"), "Accessors:Name"=w524) -> (reference out=w523:refnum<class "TTLControlledDevice.lvclass">)  [unwired: 1 in, 1 out]
            n195 = Insert Into Array(array=w526, index=w522, new element=w523) -> (w519:refnum<class "TTLControlledDevice.lvclass">[])
            n196 = Array Size(array=w519) -> (size(s)=w521:i32)
            n197 = while {
              shift-right: [w535] -> _
              shift-left: w522 -> [w527]
              tunnel: w521 -> [w531]
              tunnel: w520 -> [w533]
              tunnel: w519 -> [w532]
              stop <- w534 stop-if-true
              n198 = Index Array(array=w533, index=w527) -> (element=w530:refnum<vi>)
              n199 = Index Array(array=w532, index=w527) -> (element=w529:refnum<class "TTLControlledDevice.lvclass">)
              n200 = property class="TTLDeviceCtl (strict)"(reference=w530, "Value"=w529, "Visible"=TRUE) -> ()  [unwired: 1 in, 2 out]
              n201 = Increment(x=w527) -> (x+1=w535:i32)
              n202 = Equal?(x=w535, y=w531) -> (x = y?=w534:bool)
            }
          }
          frame "Delete" {
            n203 = Delete From Array(array=w541, length=1, index=w540) -> (array with subset deleted=w537:refnum<class "TTLControlledDevice.lvclass">[])  [unwired: 1 out]
            n204 = Array Size(array=w537) -> (size(s)=w536:i32)
            n205 = for {
              tunnel: w538 -> [w544] mode=indexing
              tunnel: w536 -> [w546]
              tunnel: w537 -> [w542]
              i -> [w543]
              n206 = Less?(x=w543, y=w546) -> (x < y?=w545:bool)
              n207 = case shown="True" w545 {
                tunnel: w544 -> [w548 w553]
                tunnel: w543 -> [_ w552]
                tunnel: w542 -> [_ w551]
                frame False {
                  n208 = property class="TTLDeviceCtl (strict)"(reference=w548, "Visible"=FALSE) -> ()  [unwired: 1 in, 2 out]
                }
                frame True {
                  n209 = Index Array(array=w551, index=w552) -> (element=w549:refnum<class "TTLControlledDevice.lvclass">)
                  n210 = property class="TTLDeviceCtl (strict)"(reference=w553, "Value"=w549, "Visible"=TRUE) -> ()  [unwired: 1 in, 2 out]
                }
              }
            }
          }
          frame "Move" {
            n211 = Delete From Array(array=w561, length=1, index=w559) -> (deleted portion=w555:refnum<class "TTLControlledDevice.lvclass">[], array with subset deleted=w556:refnum<class "TTLControlledDevice.lvclass">[])
            n212 = Insert Into Array(array=w556, index=w554, new element=w555) -> (w557:refnum<class "TTLControlledDevice.lvclass">[])
            n213 = for {
              tunnel: w560 -> [w563] mode=indexing
              tunnel: w557 -> [w562] mode=indexing
              n214 = property class="TTLDeviceCtl (strict)"(reference=w563, "Value"=w562) -> ()  [unwired: 1 in, 2 out]
            }
          }
          frame "Edit" {
            n215 = Index Array(array=w566, index=w565) -> (element=w564:refnum<class "TTLControlledDevice.lvclass">)
            n216 = property class="TTLDevice"(reference=w564, "Accessors:Name"=w573) -> (reference out=w572:refnum<class "TTLControlledDevice.lvclass">)  [unwired: 1 in, 1 out]
            n217 = Replace Array Subset(array=w566, new element=w572, index=w565) -> (w570:refnum<class "TTLControlledDevice.lvclass">[])
            n218 = Index Array(array=w571, index=w565) -> (element=w569:refnum<vi>)
            n219 = Index Array(array=w570, index=w565) -> (element=w568:refnum<class "TTLControlledDevice.lvclass">)
            n220 = property class="TTLDeviceCtl (strict)"(reference=w569, "Value"=w568, "Visible"=TRUE) -> ()  [unwired: 1 in, 2 out]
          }
        }
      }
      event "DigDevice 0", "DigDevice 1", "DigDevice 2", "DigDevice 3", "DigDevice 4": Value Change {
        n221 = event-data() -> ("NewVal"=w577:refnum<class "TTLControlledDevice.lvclass">, "CtlRef"=w579:refnum<vi>)  [unwired: 1 in]
        n222 = Search 1D Array(1D array=w580, element=w579) -> (index of element=w576:i32)  [unwired: 1 in]
        n223 = Replace Array Subset(array=w581, new element=w577, index=w576) -> (w578:refnum<class "TTLControlledDevice.lvclass">[])
      }
    }
  }
  "Changed" <- w10
  n224 = Unregister For Events(event registration refnum=w11) -> ()  [unwired: 1 in, 1 out]
